vi "Leap Motion - Pinch shape data.vi"(8 "Error In":errorcluster, 10 "Pinch":bool[](array[boolean])) -> (0 "Error Out":errorcluster, 2 "Pinch cluster":T1)   [LabVIEW 2014]
uses:
  Typedef/pinch_data.ctl
panel:
  in  "Pinch data":T1
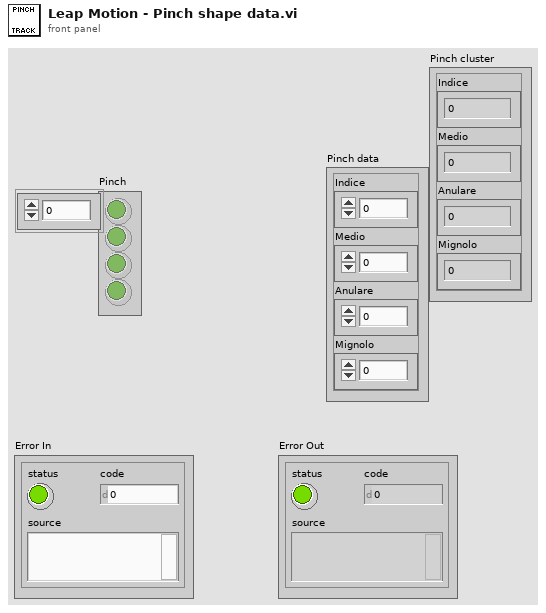
[diagram p1: front panel]
types:
  T1 = typedef "pinch_data.ctl" = cluster{"Indice":u8, "Medio":u8, "Anulare":u8, "Mignolo":u8}
  T2 = cluster{"Pinch[0]":bool, "Pinch[1]":bool, "Pinch[2]":bool, "Pinch[3]":bool, "Pinch[4]":bool}
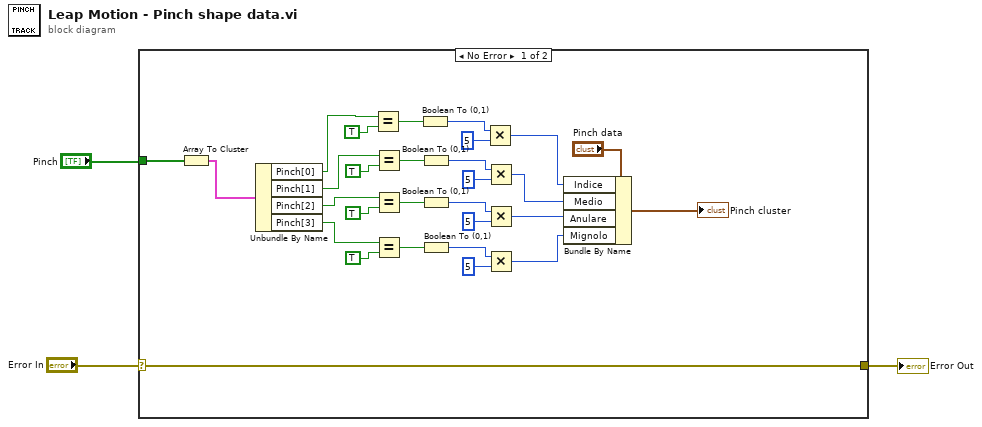
[diagram p0: block diagram]
diagram:
  n1 = case shown="No Error" "Error In" {
    selector: "Error In" -> [w32 w33]
    tunnel: [w32 w33] -> w2
    tunnel: "Pinch" -> [w31 _]
    frame No Error {
      n2 = Array To Cluster(array=w31) -> (cluster=w30:T2)
      n3 = Unbundle By Name(w30) -> ("Pinch[0]"=w25:bool, "Pinch[1]"=w18:bool, "Pinch[2]"=w13:bool, "Pinch[3]"=w6:bool)
      n4 = Equal?(x=w25, y=TRUE) -> (x = y?=w28:bool)
      n5 = Equal?(x=w18, y=TRUE) -> (x = y?=w21:bool)
      n6 = Equal?(x=w13, y=TRUE) -> (x = y?=w16:bool)
      n7 = Equal?(x=w6, y=TRUE) -> (x = y?=w9:bool)
      n8 = Boolean To (0,1)(Boolean=w28) -> (0, 1=w27:i16)
      n9 = Boolean To (0,1)(Boolean=w21) -> (0, 1=w20:i16)
      n10 = Boolean To (0,1)(Boolean=w16) -> (0, 1=w15:i16)
      n11 = Boolean To (0,1)(Boolean=w9) -> (0, 1=w8:i16)
      n12 = Multiply(x=w27, y=i16 5) -> (x*y=w23:i16)
      n13 = Multiply(x=w20, y=i16 5) -> (x*y=w12:i16)
      n14 = Multiply(x=w15, y=i16 5) -> (x*y=w11:i16)
      n15 = Multiply(x=w8, y=i16 5) -> (x*y=w5:i16)
      n16 = Bundle By Name(cluster="Pinch data", "Indice"=w23, "Medio"=w12, "Anulare"=w11, "Mignolo"=w5) -> (→"Pinch cluster":T1)
    }
    frame Error {
    }
  }
  "Error Out" <- w2
